vi "dot_selector.vi"(2 "n° digitos display":i32, 3 "decimal length":i32) -> (7 "dot":bool[](array[boolean]))   [LabVIEW 2025]
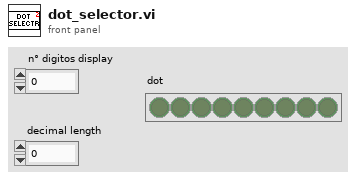
[diagram p1: front panel]
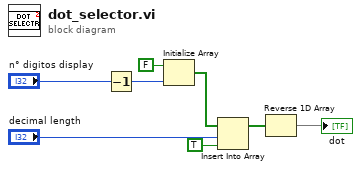
[diagram p0: block diagram]
diagram:
  n1 = Decrement(x="n° digitos display") -> (x-1=w2:i32)
  n2 = Initialize Array(FALSE, w2) -> (w3:bool[])
  n3 = Insert Into Array(array=w3, index="decimal length", new element=TRUE ("new element/subarray")) -> (w6:bool[])
  n4 = Reverse 1D Array(array=w6) -> (reversed array=→"dot":bool[])
